vi "Bullseye.vi"(9 "Color":u32(colorbox)=15688704, 10 "SizeAndLocation":T1={"X Offset"=10, "Y Offset"=170, "Height"=300, "Width"=10}, 11 "Image in":T2) -> (1 "Center":dbl, 3 "Image out":T2)   [LabVIEW 2015]
uses:
  <vilib>/vision/Image Controls.llb/IMAQ Image.ctl
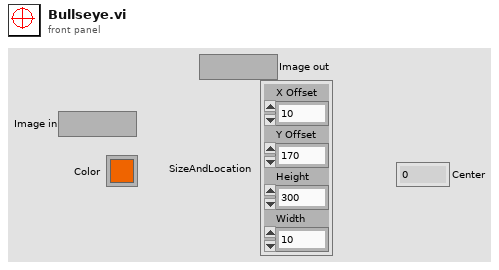
[diagram p1: front panel]
types:
  T1 = cluster{"X Offset":i32, "Y Offset":i32, "Height":i32, "Width":i32}
  T2 = typedef "IMAQ Image.ctl" = refnum<image>
  T3 = cluster{"Left":i32, "Top":i32, "Right":i32, "Bottom":i32}
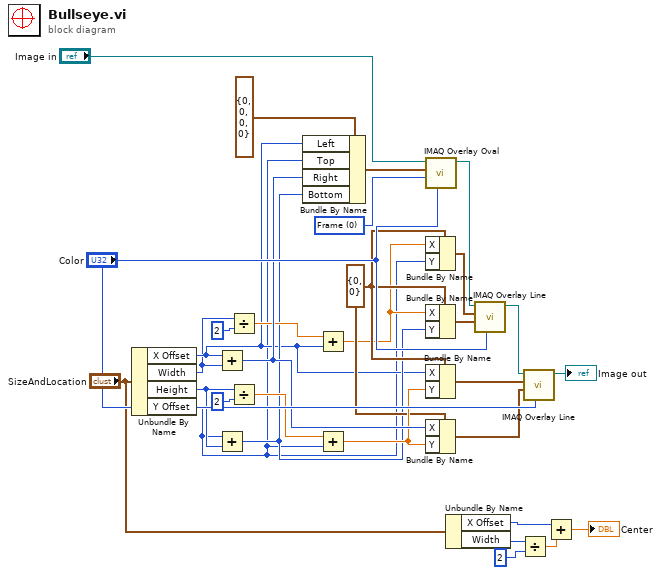
[diagram p0: block diagram]
diagram:
  w26 = cluster{"X":i32, "Y":i32} {"X"=0, "Y"=0} ("End Point")
  w12 = u32 0 items=["Frame", "Fill"] ("Drawing Mode (Frame)")
  n1 = Unbundle By Name("SizeAndLocation") -> ("X Offset"=w10:i32, "Width"=w9:i32, "Height"=w8:i32, "Y Offset"=w7:i32)
  n2 = Add(x=w10, y=w9) -> (x+y=w30:i32)
  n3 = Add(x=w7, y=w8) -> (x+y=w17:i32)
  n4 = Divide(x=w9, y=2) -> (x/y=w19:dbl)
  n5 = Divide(x=w8, y=2) -> (x/y=w27:dbl)
  n6 = Bundle By Name(cluster=T3 {"Left"=0, "Top"=0, "Right"=0, "Bottom"=0} ("Bounding Rectangle"), "Left"=w10, "Top"=w7, "Right"=w30, "Bottom"=w17) -> (w14:T3)
  n7 = Add(x=w19, y=w10) -> (x+y=w20:dbl)
  n8 = Add(x=w27, y=w7) -> (x+y=w29:dbl)
  n9 = call "IMAQ Overlay Oval"("Color"="Color", "Drawing Mode (Frame)"=w12, "Bounding Rectangle"=w14, "Image"="Image in") -> ("Image Out"=w15:T2)  [unwired: 6 in, 1 out]
  n10 = Bundle By Name(cluster=w26, "X"=w20, "Y"=w7) -> (w16:cluster{"X":i32, "Y":i32})
  n11 = Bundle By Name(cluster=w26, "X"=w20, "Y"=w17) -> (w21:cluster{"X":i32, "Y":i32})
  n12 = Bundle By Name(cluster=w26, "X"=w10, "Y"=w29) -> (w24:cluster{"X":i32, "Y":i32})
  n13 = Bundle By Name(cluster=w26, "X"=w30, "Y"=w29) -> (w25:cluster{"X":i32, "Y":i32})
  n14 = Unbundle By Name("SizeAndLocation") -> ("X Offset"=w3:i32, "Width"=w4:i32)
  n15 = call "IMAQ Overlay Line"("Color"="Color", "End Point"=w21, "Start Point"=w16, "Image"=w15) -> ("Image Out"=w22:T2)  [unwired: 6 in, 1 out]
  n16 = Divide(x=w4, y=2) -> (x/y=w6:dbl)
  n17 = call "IMAQ Overlay Line"("Color"="Color", "End Point"=w25, "Start Point"=w24, "Image"=w22) -> ("Image Out"=→"Image out":T2)  [unwired: 6 in, 1 out]
  n18 = Add(x=w3, y=w6) -> (x+y=→"Center":dbl)
